vi "Load inventory.vi"(8 "error in (no error)":errorcluster, 11 "User Interface in":refnum<class "User Interface.lvclass">) -> (0 "error out":errorcluster, 3 "User Interface out":refnum<class "User Interface.lvclass">)   [LabVIEW 2020, in "User Interface.lvlib" / "User Interface.lvclass"]
uses:
  User Interface.lvclass
  User Interface.lvclass/User Interface.ctl
  Paquetes Disponibles Messages/Read Services Msg/Read Services Msg.lvclass/Read Services Msg.ctl
  <vilib>/ActorFramework/Message Enqueuer/Message Enqueuer.lvclass/Message Enqueuer.ctl
  <vilib>/ActorFramework/Message Enqueuer/Enqueue.vi
  Paquetes Disponibles Messages/Read Services Msg/Read Services Msg.lvclass
  C:/Program Files (x86)/National Instruments/LabVIEW 2020/vi.lib/ActorFramework/Message/Message.lvclass
  <vilib>/Utility/config.llb/Read Key (U32).vi
  <vilib>/ActorFramework/Message Priority Queue/Priority Enqueue.vi
  <vilib>/Utility/config.llb/NI_LVConfig.lvlib
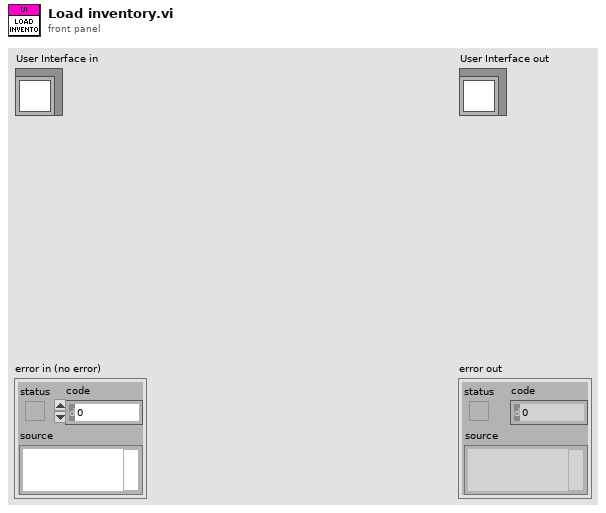
[diagram p1: front panel]
types:
  T1 = typedef "NI_LVConfig.lvlib/Config Data RefNum.ctl" = refnum<k1>
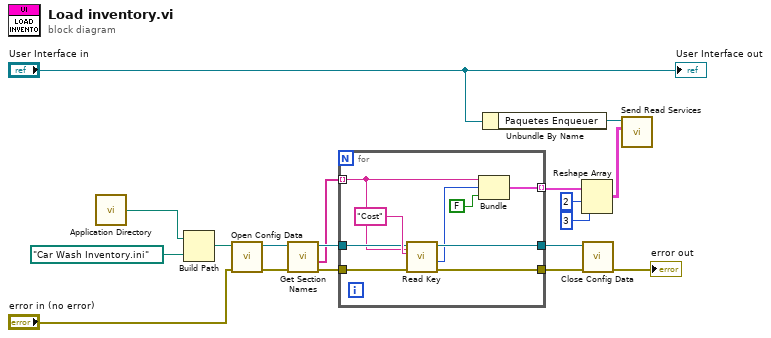
[diagram p0: block diagram]
diagram:
  n1 = call <vilib>:"Application Directory.vi"() -> ("Application Directory"=w18:path)
  n2 = Build Path(base path=w18, name or relative path=path "Car Wash Inventory.ini") -> (appended path=w15:path)
  n3 = call <vilib>:"Open Config Data.vi"("error in (no error)"="error in (no error)", "configuration file path"=w15) -> ("error out"=w16:errorcluster, "refnum"=w10:T1)  [unwired: 7 in, 1 out]
  n4 = call <vilib>:"Get Section Names.vi"("error in (no error)"=w16, "refnum"=w10) -> ("error out"=w14:errorcluster, "section names"=w9:string[], "refnum out"=w11:T1)  [unwired: 7 in]
  n5 = for {
    tunnel: w14 -> [w27]
    tunnel: [w26] -> w13
    tunnel: [w24] -> w12
    tunnel: w11 -> [w23]
    tunnel: [w20] -> _ mode=indexing
    tunnel: w9 -> [w20] mode=indexing
    tunnel: [w21] -> w8 mode=indexing
    n6 = call-poly <vilib>:"Read Key.vi"("section"=w20, "error in (no error)"=w27, "key"="Cost", "refnum"=w23) -> ("error out"=w26:errorcluster, "value"=w22:u32, "refnum out"=w24:T1)  [unwired: 4 in, 1 out]
    n7 = Bundle("String"=w20, "value"=w22, FALSE) -> (w21:cluster{"String":string, "value":u32, bool})  [unwired: 1 in]
  }
  n8 = Unbundle By Name("User Interface in") -> ("Paquetes Enqueuer"=w2:refnum<class "Message Enqueuer.lvclass">)
  n9 = Reshape Array(w8, 2 ("dimension size"), 3 ("dimension size")) -> (w1:cluster{"String":string, "value":u32, bool}[][])
  n10 = call <vilib>:"Close Config Data.vi"("error in (no error)"=w13, "refnum"=w12) -> ("error out"=→"error out":errorcluster)  [unwired: 8 in, 1 out]
  n11 = call "Send Read Services.vi"("Wash Car Cost"=w1, "Message Enqueuer"=w2) -> ()  [unwired: 8 in, 2 out]
  "User Interface out" <- "User Interface in"
